vi "Check Network Connection.vi"(9 "CD Path":string, 10 "IP Address":string, 11 "connection info":T1) -> (0 "error out":errorcluster, 3 "connection info":T1)   [LabVIEW 2019, in "Instrument Workspace Objects.lvlib"]
uses:
  Instrument Workspace Objects.lvlib
  <vilib>/NI/STM/TCP/TCP Connection Info.ctl
  <vilib>/NI/STM/SubVIs/MetaDataElement.ctl
  Host API/Instrument CD Host API.lvlib
  <vilib>/NI/STM/NI STM.lvlib
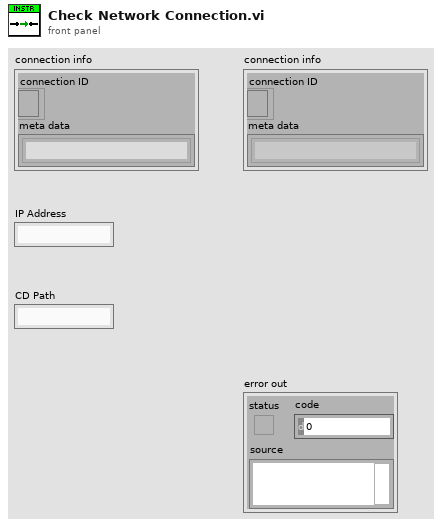
[diagram p1: front panel]
types:
  T1 = typedef "NI STM.lvlib/TCP Connection Info.ctl" = cluster{"connection ID":refnum<k5>, "meta data":T2[]}
  T2 = typedef "NI STM.lvlib/MetaDataElement.ctl" = string
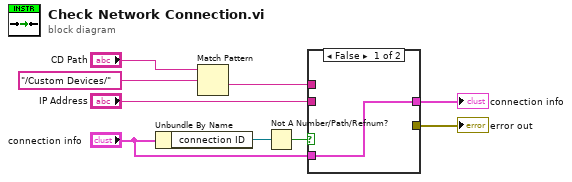
[diagram p0: block diagram]
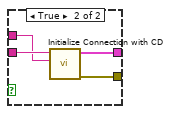
[diagram p2: hidden frame]
diagram:
  n1 = Unbundle By Name("connection info") -> ("connection ID"=w4:refnum<k5>)
  n2 = Match Pattern(string="CD Path", regular expression="/Custom Devices/" ("Custom Device Path")) -> (after substring=w1:string)  [unwired: 1 in, 3 out]
  n3 = Not A Number/Path/Refnum?(number/path/refnum=w4) -> (NaN/Path/Refnum?=w8:bool)
  n4 = case shown="False" w8 {
    tunnel: w1 -> [_ w13]
    tunnel: [w10 w11] -> w6
    tunnel: "connection info" -> [w10 _]
    tunnel: [_ w12] -> w9
    tunnel: "IP Address" -> [_ w14]
    frame False {
    }
    frame True {
      n5 = call "Initialize Connection with CD.vi"("TCP Service"=w13, "IP Address"=w14) -> ("error out"=w12:errorcluster, "connection info out"=w11:T1)  [unwired: 8 in]
    }
  }
  "error out" <- w9
  "connection info" <- w6
